vi "Init Hardware.vi"(8 "error in (no error)":errorcluster, 11 "Signal Recovery Driver in":refnum<class "Signal Recovery Driver.lvclass">) -> (0 "error out":errorcluster, 3 "Signal Recovery Driver out":refnum<class "Signal Recovery Driver.lvclass">)   [LabVIEW 2025, in "Signal Recovery Driver.lvclass"]
uses:
  Signal Recovery Driver.lvclass
  C:/GitHub/NHMFL_Core/Libraries/Instruments/Instrument Driver/Instrument Driver.lvclass
  Instrument Driver/Instrument Driver.lvclass/Instrument Driver.ctl
  Instrument Driver/Read Recorder name.vi
  Instrument Driver/Write Channel names.vi
  Instrument Driver/Write Channel units.vi
  Simple VISA Reader/Simple VISA Reader Driver.lvclass
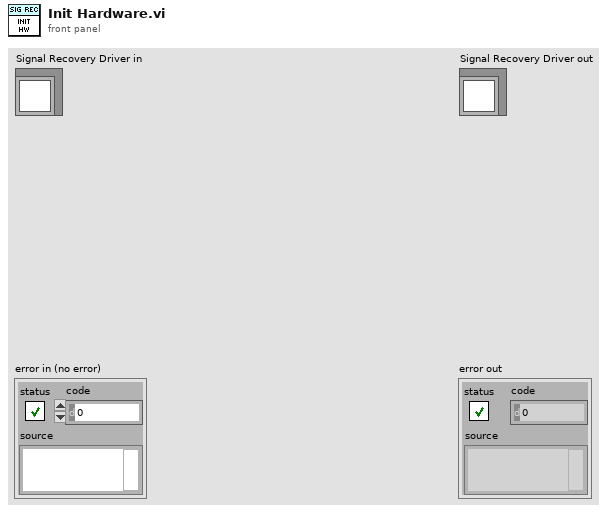
[diagram p1: front panel]
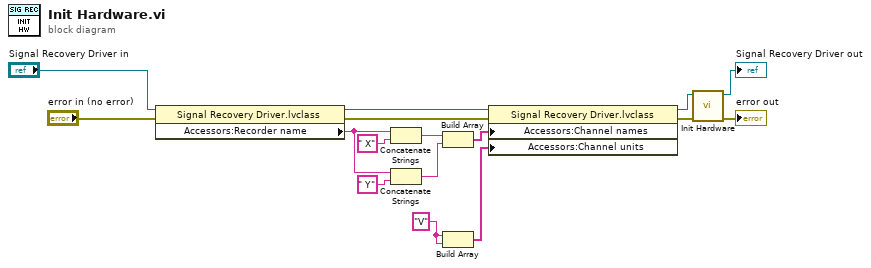
[diagram p0: block diagram]
diagram:
  w5 = "V"
  n1 = property class="Signal Recovery Driver.lvclass"(reference="Signal Recovery Driver in", error in="error in (no error)") -> (reference out=w13:refnum<class "Signal Recovery Driver.lvclass">, error out=w14:errorcluster, "Accessors:Recorder name"=w8:string)
  n2 = Concatenate Strings(w8, " X") -> (w9:string)
  n3 = Concatenate Strings(w8, " Y") -> (w6:string)
  n4 = Build Array(w9, w6) -> (w11:string[])
  n5 = Build Array(w5, w5) -> (w12:string[])
  n6 = property class="Signal Recovery Driver.lvclass"(reference=w13, error in=w14, "Accessors:Channel names"=w11, "Accessors:Channel units"=w12) -> (reference out=w1:refnum<class "Signal Recovery Driver.lvclass">, error out=w2:errorcluster)
  n7 = call-parent "Init Hardware.vi"("error in (no error)"=w2, "Instrument Driver in"=w1) -> ("error out"=→"error out":errorcluster, "Instrument Driver out"=→"Signal Recovery Driver out":refnum<class "Signal Recovery Driver.lvclass">)  [unwired: 8 in]
